vi "Challenge UI.vi"() -> ()   [LabVIEW 2024]
uses:
  <vilib>/Utility/miscctls.llb/LVRectTypeDef.ctl
panel:
  out "0 2":bool
  out "0 3":bool
  out "0 4":bool
  out "0 5":bool
  out "0 6":bool
  out "0 7":bool
  out "0 8":bool
  out "0 9":bool
  out "0 10":bool
  out "0 11":bool
  out "0 12":bool
  out "0 13":bool
  out "0 14":bool
  out "0 15":bool
  out "0 16":bool
  out "0 17":bool
  out "0 18":bool
  out "0 19":bool
  out "0 20":bool
  out "0 21":bool
  out "0 22":bool
  out "0 23":bool
  out "0 24":bool
  out "0 25":bool
  out "0 26":bool
  in  "Stop":bool
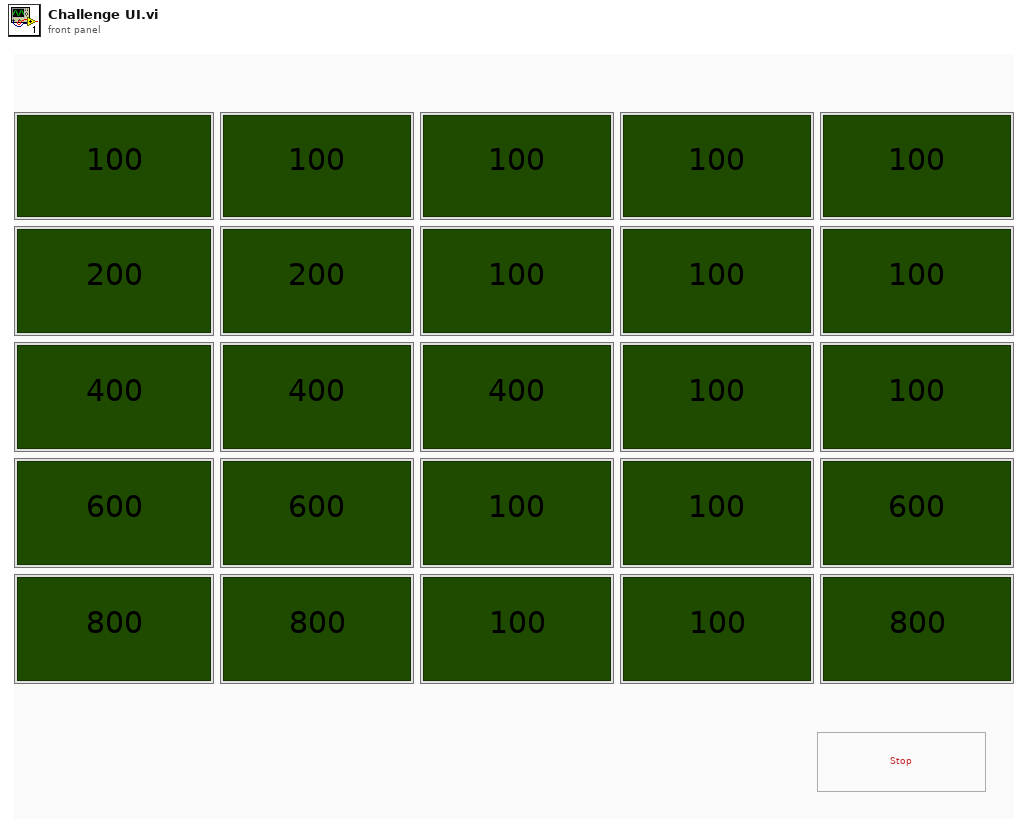
[diagram p1: front panel]
types:
  T1 = enum16{"Sticks Top/Left", "Sticks Bottom/Right", "Proportional"}
  T2 = typedef "LVRectTypeDef.ctl" = cluster{"Left":i16, "Top":i16, "Right":i16, "Bottom":i16}
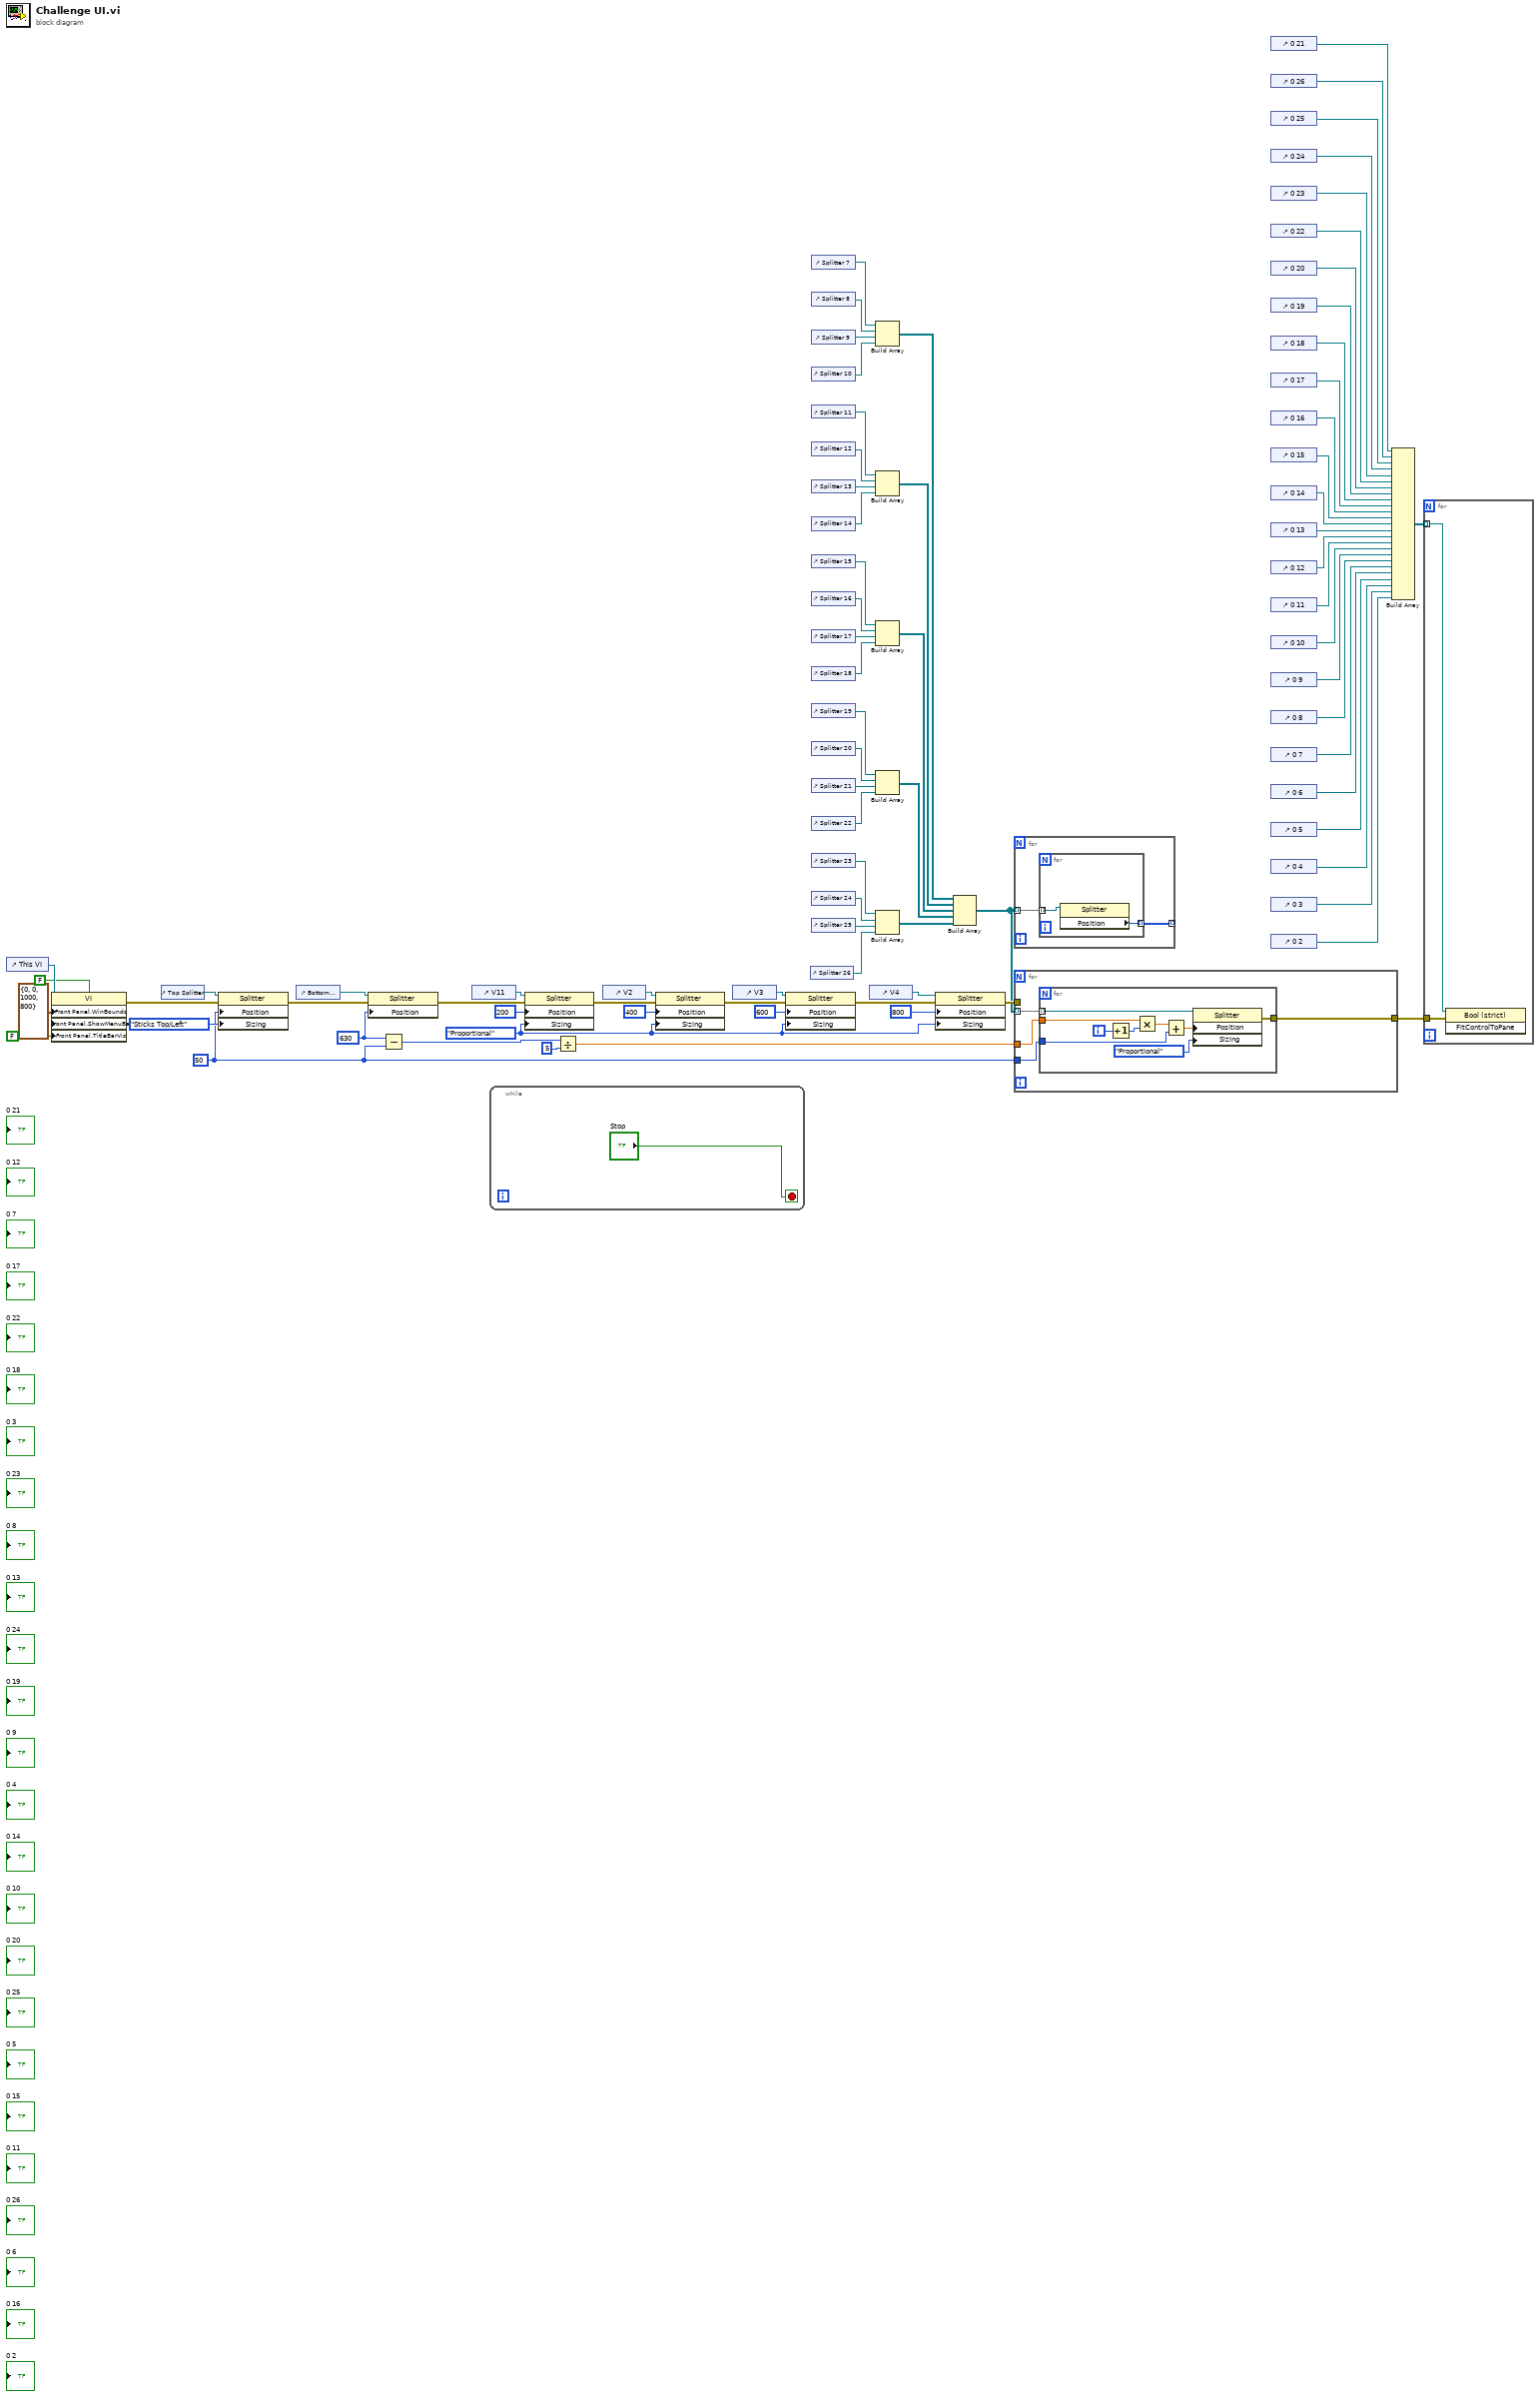
[diagram p0: block diagram]
diagram:
  w67 = T1."Proportional" ("Sizing")
  w34 = 630 ("Splitter Position")
  w33 = 50 ("Splitter Position")
  n1 = control-ref of="This VI"() -> (w80:refnum<vi>)
  n2 = property class="VI"(reference=w80, "Front Panel.WinBounds"=T2 {"Left"=0, "Top"=0, "Right"=1000, "Bottom"=800} ("Front Panel Window:Window Bounds"), "Front Panel.ShowMenuBar"=FALSE ("Front Panel Window:Show Menu Bar"), "Front Panel.TitleBarVis"=FALSE ("Front Panel Window:Title Bar Visible")) -> (error out=w77:errorcluster)  [unwired: 1 in, 1 out]
  n3 = control-ref of="Top Splitter"() -> (w79:refnum<vi>)
  n4 = property class="Splitter"(reference=w79, error in=w77, "Position"=w33, "Sizing"=T1."Sticks Top/Left") -> (error out=w76:errorcluster)  [unwired: 1 out]
  n5 = control-ref of="Bottom Splitter"() -> (w78:refnum<vi>)
  n6 = property class="Splitter"(reference=w78, error in=w76, "Position"=w34) -> (error out=w62:errorcluster)  [unwired: 1 out]
  n7 = Subtract(x=w34, y=w33) -> (x-y=w32:i32)
  n8 = control-ref of="V11"() -> (w74:refnum<vi>)
  n9 = while {
    stop <- "Stop" stop-if-true
  }
  n10 = property class="Splitter"(reference=w74, error in=w62, "Position"=200 ("Splitter Position"), "Sizing"=w67) -> (error out=w65:errorcluster)  [unwired: 1 out]
  n11 = Divide(x=w32, y=5) -> (x/y=w30:dbl)
  n12 = control-ref of="V2"() -> (w72:refnum<vi>)
  n13 = property class="Splitter"(reference=w72, error in=w65, "Position"=400 ("Splitter Position"), "Sizing"=w67) -> (error out=w64:errorcluster)  [unwired: 1 out]
  n14 = control-ref of="V3"() -> (w70:refnum<vi>)
  n15 = property class="Splitter"(reference=w70, error in=w64, "Position"=600 ("Splitter Position"), "Sizing"=w67) -> (error out=w63:errorcluster)  [unwired: 1 out]
  n16 = control-ref of="Splitter 26"() -> (w46:refnum<vi>)
  n17 = control-ref of="Splitter 7"() -> (w61:refnum<vi>)
  n18 = control-ref of="Splitter 8"() -> (w60:refnum<vi>)
  n19 = control-ref of="Splitter 9"() -> (w59:refnum<vi>)
  n20 = control-ref of="Splitter 10"() -> (w58:refnum<vi>)
  n21 = control-ref of="Splitter 11"() -> (w57:refnum<vi>)
  n22 = control-ref of="Splitter 12"() -> (w56:refnum<vi>)
  n23 = control-ref of="Splitter 13"() -> (w43:refnum<vi>)
  n24 = control-ref of="Splitter 14"() -> (w42:refnum<vi>)
  n25 = control-ref of="Splitter 15"() -> (w55:refnum<vi>)
  n26 = control-ref of="Splitter 16"() -> (w44:refnum<vi>)
  n27 = control-ref of="Splitter 17"() -> (w54:refnum<vi>)
  n28 = control-ref of="Splitter 18"() -> (w53:refnum<vi>)
  n29 = control-ref of="Splitter 19"() -> (w45:refnum<vi>)
  n30 = control-ref of="Splitter 20"() -> (w52:refnum<vi>)
  n31 = control-ref of="Splitter 21"() -> (w51:refnum<vi>)
  n32 = control-ref of="Splitter 22"() -> (w50:refnum<vi>)
  n33 = control-ref of="Splitter 23"() -> (w49:refnum<vi>)
  n34 = control-ref of="Splitter 24"() -> (w48:refnum<vi>)
  n35 = control-ref of="Splitter 25"() -> (w47:refnum<vi>)
  n36 = control-ref of="V4"() -> (w68:refnum<vi>)
  n37 = Build Array(w61, w60, w59, w58) -> (w41:refnum<vi>[])
  n38 = Build Array(w57, w56, w43, w42) -> (w40:refnum<vi>[])
  n39 = Build Array(w55, w44, w54, w53) -> (w39:refnum<vi>[])
  n40 = Build Array(w45, w52, w51, w50) -> (w38:refnum<vi>[])
  n41 = Build Array(w49, w48, w47, w46) -> (w37:refnum<vi>[])
  n42 = property class="Splitter"(reference=w68, error in=w63, "Position"=800 ("Splitter Position"), "Sizing"=w67) -> (error out=w36:errorcluster)  [unwired: 1 out]
  n43 = Build Array(w41, w40, w39, w38, w37) -> (w35:refnum<vi>[][])
  n44 = for {
    tunnel: w35 -> [w84] mode=indexing
    tunnel: [w83] -> _ mode=indexing
    n45 = for {
      tunnel: w84 -> [w86] mode=indexing
      tunnel: [w85] -> w83 mode=indexing
      n46 = property class="Splitter"(reference=w86) -> ("Position"=w85:i32)  [unwired: 1 in, 2 out]
    }
  }
  n47 = for {
    tunnel: w35 -> [w90] mode=indexing
    tunnel: w36 -> [_]
    tunnel: [w89] -> w3
    tunnel: w33 -> [w88]
    tunnel: w30 -> [w87]
    n48 = for {
      tunnel: w90 -> [w99] mode=indexing
      tunnel: [w95] -> w89
      tunnel: w88 -> [w92]
      tunnel: w87 -> [w91]
      i -> [w98]
      n49 = Increment(x=w98) -> (x+1=w96:i32)
      n50 = Multiply(x=w91, y=w96) -> (x*y=w94:dbl)
      n51 = Add(x=w94, y=w92) -> (x+y=w93:dbl)
      n52 = property class="Splitter"(reference=w99, "Position"=w93, "Sizing"=T1."Proportional") -> (error out=w95:errorcluster)  [unwired: 1 in, 1 out]
    }
  }
  n53 = control-ref of="0 21"() -> (w4:refnum<vi>)
  n54 = control-ref of="0 26"() -> (w29:refnum<vi>)
  n55 = control-ref of="0 25"() -> (w28:refnum<vi>)
  n56 = control-ref of="0 24"() -> (w27:refnum<vi>)
  n57 = control-ref of="0 23"() -> (w26:refnum<vi>)
  n58 = control-ref of="0 22"() -> (w25:refnum<vi>)
  n59 = control-ref of="0 20"() -> (w24:refnum<vi>)
  n60 = control-ref of="0 19"() -> (w23:refnum<vi>)
  n61 = control-ref of="0 18"() -> (w22:refnum<vi>)
  n62 = control-ref of="0 17"() -> (w21:refnum<vi>)
  n63 = control-ref of="0 16"() -> (w20:refnum<vi>)
  n64 = control-ref of="0 15"() -> (w19:refnum<vi>)
  n65 = control-ref of="0 14"() -> (w18:refnum<vi>)
  n66 = control-ref of="0 13"() -> (w17:refnum<vi>)
  n67 = control-ref of="0 12"() -> (w16:refnum<vi>)
  n68 = control-ref of="0 11"() -> (w15:refnum<vi>)
  n69 = control-ref of="0 10"() -> (w14:refnum<vi>)
  n70 = control-ref of="0 9"() -> (w13:refnum<vi>)
  n71 = control-ref of="0 8"() -> (w12:refnum<vi>)
  n72 = control-ref of="0 7"() -> (w11:refnum<vi>)
  n73 = control-ref of="0 6"() -> (w10:refnum<vi>)
  n74 = control-ref of="0 5"() -> (w9:refnum<vi>)
  n75 = control-ref of="0 4"() -> (w8:refnum<vi>)
  n76 = control-ref of="0 3"() -> (w7:refnum<vi>)
  n77 = control-ref of="0 2"() -> (w6:refnum<vi>)
  n78 = Build Array(w4, w29, w28, w27, w26, w25, w24, w23, w22, w21, w20, w19, w18, w17, w16, w15, w14, w13, w12, w11, w10, w9, w8, w7, w6) -> (w5:refnum<vi>[])
  n79 = for {
    tunnel: w5 -> [w101] mode=indexing
    tunnel: w3 -> [w100]
    n80 = invoke class="Bool (strict)" method="FitControlToPane"(reference=w101, error in=w100) -> ()  [unwired: 1 in, 3 out]
  }
